vi "Final-Initial Slope.vi"(2 "X Array":dbl[](array[numeric]) format="%.2f", 3 "Y Array":dbl[](array[numeric]) format="%.2f") -> (0 "Final Slope":dbl format="%.2f", 1 "Initial Slope":dbl format="%.2f")   [LabVIEW 2019]
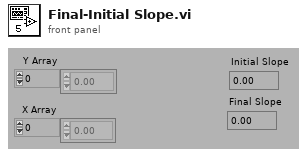
[diagram p1: front panel]
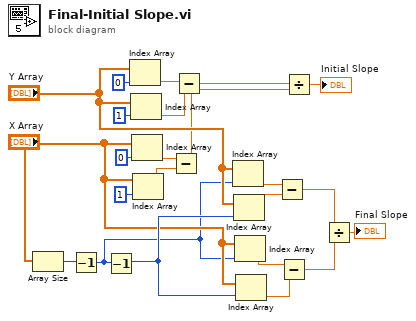
[diagram p0: block diagram]
diagram:
  n1 = Array Size(array="X Array") -> (size(s)=w19:i32)
  n2 = Decrement(x=w19) -> (x-1=w1:i32)
  n3 = Decrement(x=w1) -> (x-1=w18:i32)
  n4 = Index Array(array="Y Array", index=0) -> (element=w15:dbl)
  n5 = Index Array(array="Y Array", index=1) -> (element=w14:dbl)
  n6 = Index Array(array="X Array", index=0) -> (element=w13:dbl)
  n7 = Index Array(array="X Array", index=1) -> (element=w12:dbl)
  n8 = Subtract(x=w13, y=w12) -> (x-y=w10:dbl)
  n9 = Subtract(x=w15, y=w14) -> (x-y=w11:dbl)
  n10 = Index Array(array="Y Array", index=w1) -> (element=w9:dbl)
  n11 = Index Array(array="Y Array", index=w18) -> (element=w8:dbl)
  n12 = Index Array(array="X Array", index=w1) -> (element=w7:dbl)
  n13 = Index Array(array="X Array", index=w18) -> (element=w6:dbl)
  n14 = Subtract(x=w9, y=w8) -> (x-y=w4:dbl)
  n15 = Subtract(x=w7, y=w6) -> (x-y=w5:dbl)
  n16 = Divide(x=w11, y=w10) -> (x/y=→"Initial Slope":dbl)
  n17 = Divide(x=w4, y=w5) -> (x/y=→"Final Slope":dbl)
